vi "Configuration Complete(subvi).vi"(8 "error in":errorcluster, 11 "FPGA VI Reference In":refnum<k20>) -> (0 "error out":errorcluster, 2 "Configured?":bool, 3 "FPGA VI Reference Out":refnum<k20>)   [LabVIEW 2015]
uses:
  <vilib>/Utility/error.llb/Error Cluster From Error Code.vi
  <vilib>/rvi/errors/niLvFpgaAdjustHostInterfaceError.vi
  <vilib>/rvi/interface/nirviReadWriteControl/nirviReadWriteControl.xnode
  NiFpgaLv.dll
  <vilib>/rvi/interface/Simulation/niFpgaSimulationCallBeginRW.vi
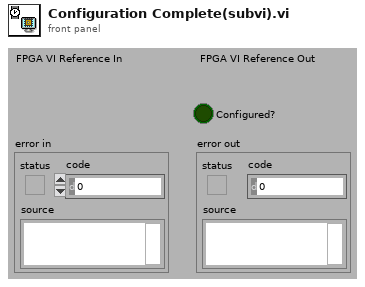
[diagram p1: front panel]
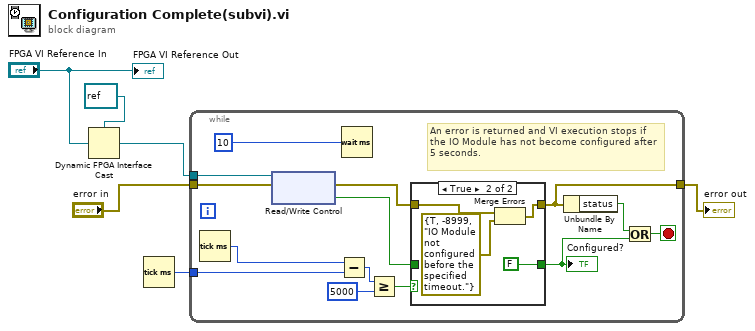
[diagram p0: block diagram]
diagram:
  n1 = Dynamic FPGA Interface Cast(Session In=refnum<k20> refnum ("FPGA VI Reference Out"), Type="FPGA VI Reference In") -> (Session Out=w3:refnum<k20>)
  n2 = Tick Count (ms)() -> (millisecond timer value=w4:u32)
  n3 = while {
    tunnel: "error in" -> [w13]
    tunnel: [w17] -> w5
    tunnel: w3 -> [w12]
    tunnel: w4 -> [w8]
    stop <- w15 stop-if-true
    # "An error is returned and VI execution stops if the IO Module has not become configured after 5 seconds."
    n4 = Tick Count (ms)() -> (millisecond timer value=w9:u32)
    n5 = xnode "Read/Write Control"("FPGA VI Reference In"=w12, "error in"=w13) -> ("error out"=w10:errorcluster, "InitDone"=w11:bool)  [unwired: 1 out]
    n6 = Subtract(x=w9, y=w8) -> (x-y=w7:u32)
    n7 = Wait (ms)(milliseconds to wait=u32 10) -> ()  [unwired: 1 out]
    n8 = Greater Or Equal?(x=w7, y=u32 5000) -> (x >= y?=w18:bool)
    n9 = case shown="True" w18 {
      tunnel: [w22 FALSE ("Configured?")] -> w14
      tunnel: w11 -> [w22 _]
      tunnel: [w21 w25] -> w17
      tunnel: w10 -> [w21 w23]
      frame False {
      }
      frame True {
        n10 = Merge Errors(w23, errorcluster {"status"=TRUE, "code"=-8999, "source"="IO Module not configured before the specified timeout."} ("error in")) -> (w25:errorcluster)
      }
    }
    "Configured?" <- w14
    n11 = Unbundle By Name(w17) -> ("status"=w16:bool)
    n12 = Or(x=w16, y=w14) -> (x .or. y?=w15:bool)
  }
  "error out" <- w5
  "FPGA VI Reference Out" <- "FPGA VI Reference In"
